vi "UI.VersionCheck.vi"(7 "path":path caption="路径", 8 "错误输入":errorcluster, 10 "Version":string="V1.0.0", 11 "App Name":string="YourAppName.exe") -> (0 "error out":errorcluster caption="错误输出", 2 "OperationCode":i8, 3 "OK?":bool)   [LabVIEW 2012, in "Lib_UEL.ATE.lvlib" / "Lib_App.lvlib"]
uses:
  Lib_App.lvlib
  <vilib>/Utility/config.llb/Read Key (String).vi
  <vilib>/Utility/config.llb/Write Key (String).vi
  <vilib>/Utility/config.llb/NI_LVConfig.lvlib
panel:
  # "OperationCode:\n-255:错误\n-1:运行的不是最新版本\n0:运行版本与版本列表一致\n1:运行版本比版本列表新, 写入最新版本到版本列表\n2:没有在版本列表找到相关版本信息"
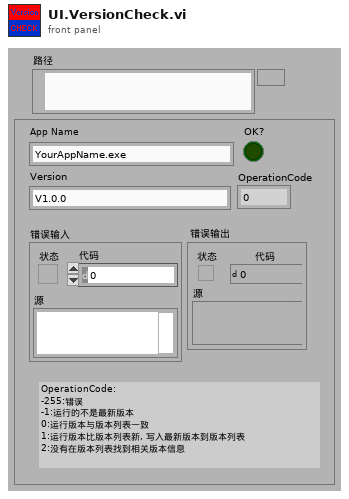
[diagram p1: front panel]
types:
  T1 = typedef "NI_LVConfig.lvlib/Config Data RefNum.ctl" = refnum<k1>
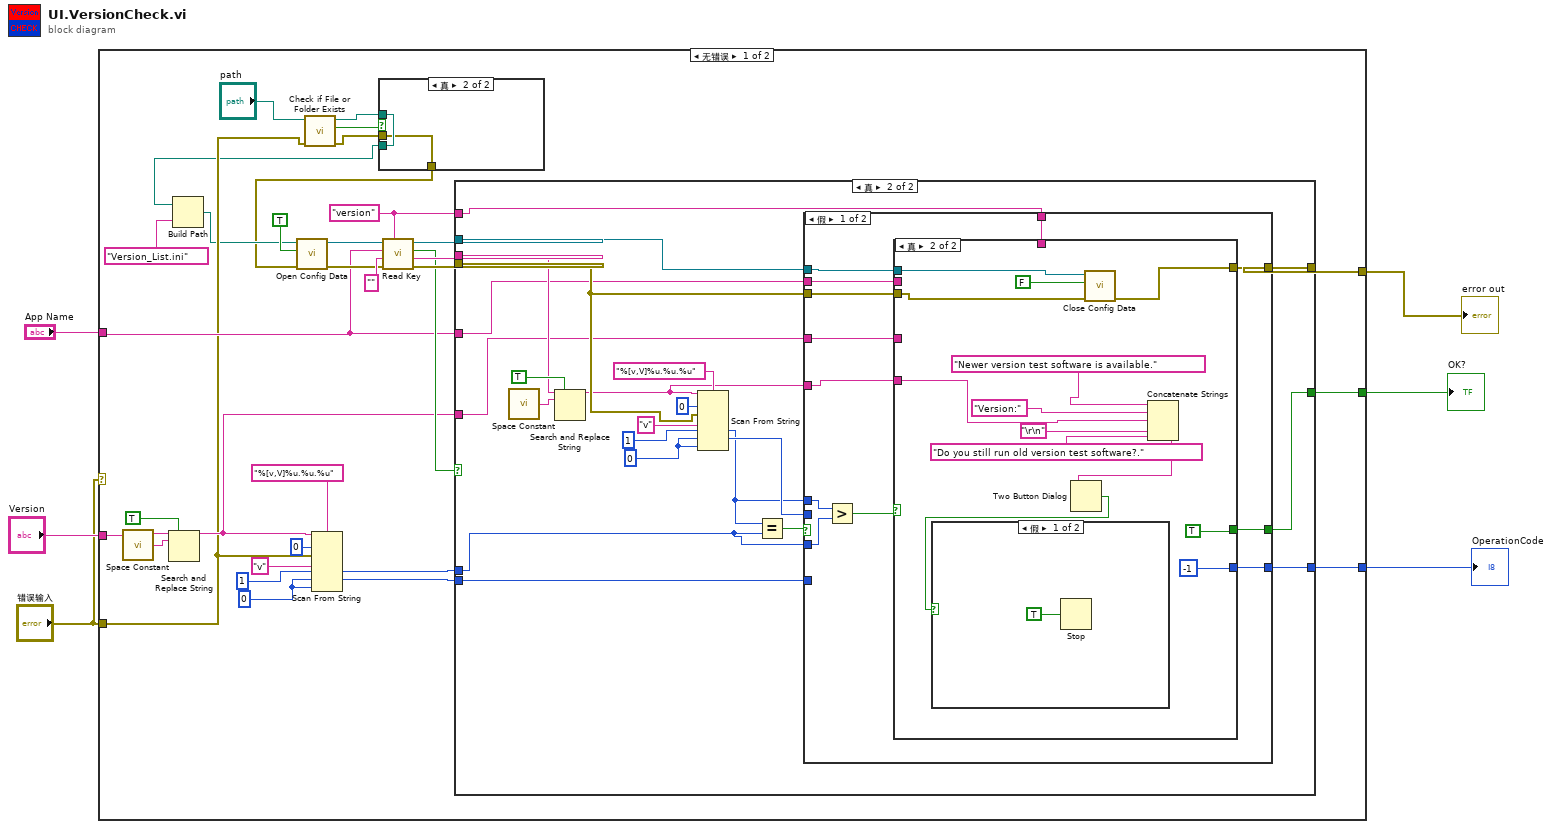
[diagram p0: block diagram]
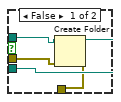
[diagram p2: hidden frame]
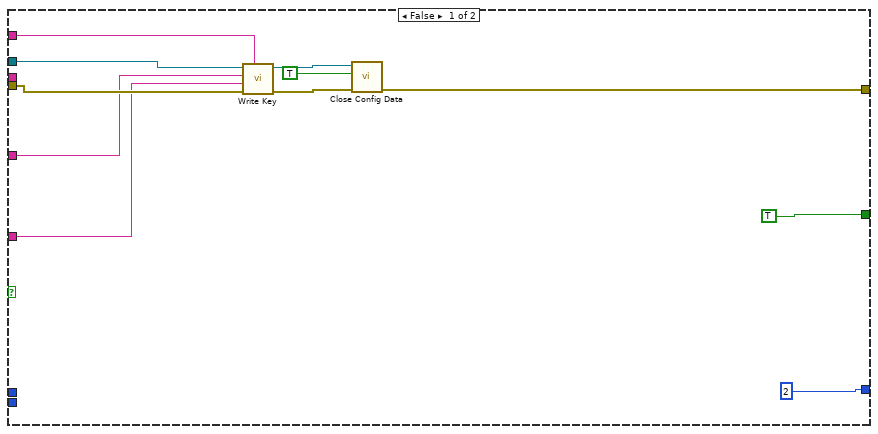
[diagram p3: hidden frame]
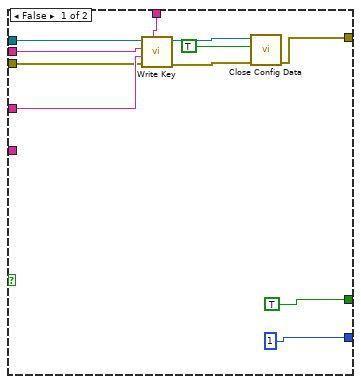
[diagram p4: hidden frame]
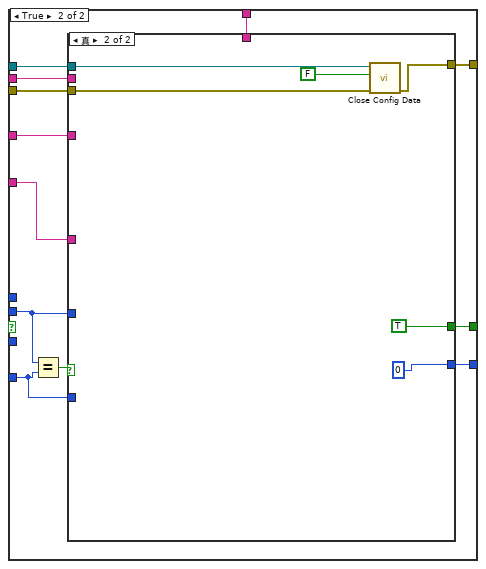
[diagram p6: hidden frame]
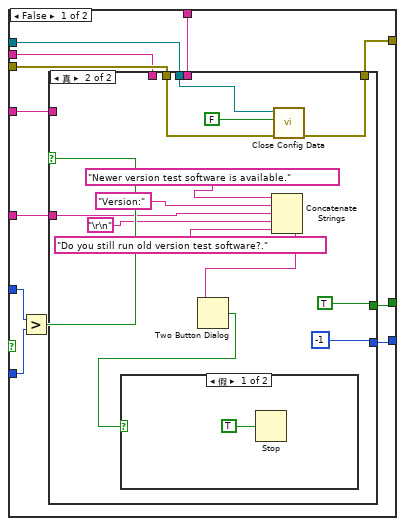
[diagram p7: hidden frame]
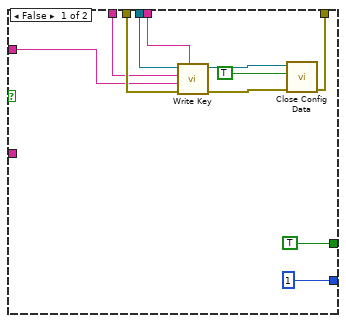
[diagram p8: hidden frame]
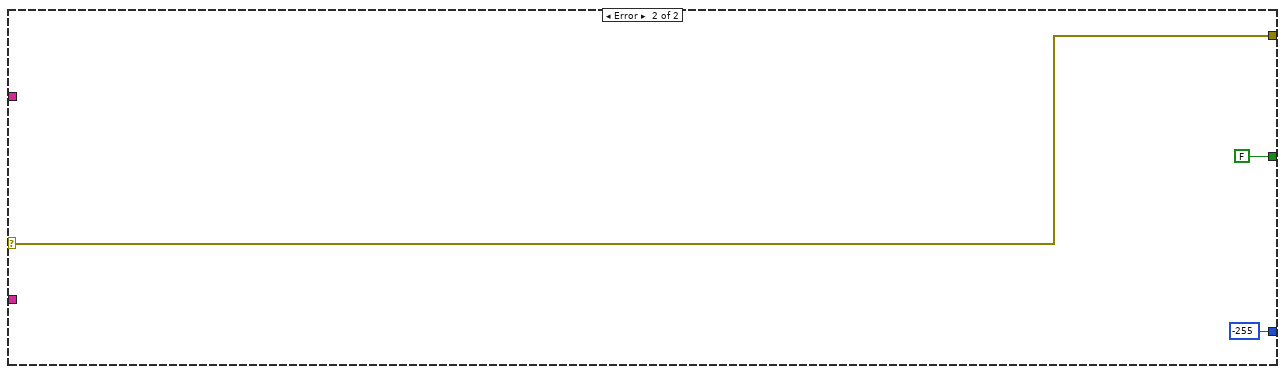
[diagram p10: hidden frame]
diagram:
  n1 = case shown="无错误" "错误输入" {
    selector: "错误输入" -> [_ w173]
    tunnel: "错误输入" -> [w13 _]
    tunnel: "Version" -> [w34 _]
    tunnel: "App Name" -> [w22 _]
    tunnel: [w24 w173] -> w3
    tunnel: [w17 -255] -> w2
    tunnel: [w16 FALSE ("OK?")] -> w1
    frame No Error {
      w20 = "version" ("section")
      w37 = 0 ("默认值 2")
      n2 = call <vilib>:"Space Constant.vi"() -> ("String"=w32:string)
      n3 = Search and Replace String(replace all?=TRUE ("替换全部？(F)"), input string=w34, search string=w32) -> (result string=w21:string)  [unwired: 5 in, 3 out]
      n4 = call <vilib>:"Check if File or Folder Exists.vi"("error in (no error)"=w13, "path"="path") -> ("error out"=w9:errorcluster, "file or folder exists?"=w15:bool, "dup path"=w14:path)  [unwired: 7 in]
      n5 = Scan From String(format string="%[v,V]%u.%u.%u" ("格式字符串"), input string=w21, initial scan location=u32 0 ("初始扫描位置"), error in=w13, default 1="v" ("默认值 1"), default 2=1 ("默认值 1"), default 3=w37, default 4=w37) -> (output 2=w19:i32, output 3=w18:i32)  [unwired: 2 in, 3 out]
      n6 = case shown="真" w15 {
        tunnel: w14 -> [w43 w45]
        tunnel: [w42 w45] -> w11
        tunnel: w9 -> [w41 w44]
        tunnel: [w40 w44] -> w8
        frame False {
          n7 = Create Folder(path (use dialog)=w43, error in=w41) -> (created path=w42:path, error out=w40:errorcluster)  [unwired: 1 in, 1 out]
        }
        frame True {
        }
      }
      n8 = Build Path(base path=w11, name or relative path="Version_List.ini" ("名称或相对路径")) -> (appended path=w10:path)
      n9 = call <vilib>:"Open Config Data.vi"("error in (no error)"=w8, "create file if necessary (T)"=TRUE ("create file if necessary? (T)"), "configuration file path"=w10) -> ("error out"=w27:errorcluster, "refnum"=w30:T1)  [unwired: 6 in, 1 out]
      n10 = call-poly <vilib>:"Read Key.vi"("section"=w20, "error in (no error)"=w27, "default value"="" ("key"), "key"=w22, "refnum"=w30) -> ("error out"=w26:errorcluster, "value"=w28:string, "found?"=w23:bool, "refnum out"=w25:T1)  [unwired: 3 in]
      n11 = case shown="真" w23 {
        tunnel: w28 -> [_ w71]
        tunnel: w26 -> [w56 w64]
        tunnel: w25 -> [w55 w65]
        tunnel: [w48 w63] -> w24
        tunnel: w22 -> [w54 w60]
        tunnel: w21 -> [w53 w61]
        tunnel: w20 -> [w52 w62]
        tunnel: w19 -> [_ w57]
        tunnel: w18 -> [_ w68]
        tunnel: [2 w67] -> w17
        tunnel: [TRUE ("OK?") w66] -> w16
        frame False {
          n12 = call-poly <vilib>:"Write Key.vi"("section"=w52, "error in (no error)"=w56, "value"=w53, "key"=w54, "refnum"=w55) -> ("error out"=w49:errorcluster, "refnum out"=w50:T1)  [unwired: 4 in, 1 out]
          n13 = call <vilib>:"Close Config Data.vi"("error in (no error)"=w49, "write file if changed (T)"=TRUE ("write configuration file? (T)"), "refnum"=w50) -> ("error out"=w48:errorcluster)  [unwired: 7 in, 1 out]
        }
        frame True {
          w74 = 0 ("默认值 2")
          n14 = call <vilib>:"Space Constant.vi"() -> ("String"=w78:string)
          n15 = Search and Replace String(replace all?=TRUE ("替换全部？(F)"), input string=w71, search string=w78) -> (result string=w59:string)  [unwired: 5 in, 3 out]
          n16 = Scan From String(format string="%[v,V]%u.%u.%u" ("格式字符串"), input string=w59, initial scan location=u32 0 ("初始扫描位置"), error in=w64, default 1="v" ("默认值 1"), default 2=1 ("默认值 1"), default 3=w74, default 4=w74) -> (output 2=w58:i32, output 3=w69:i32)  [unwired: 2 in, 3 out]
          n17 = Equal?(x=w58, y=w57) -> (x = y?=w70:bool)
          n18 = case shown="假" w70 {
            tunnel: w69 -> [_ w121]
            tunnel: w68 -> [_ w120]
            tunnel: [w80 w126] -> w67
            tunnel: [w81 w125] -> w66
            tunnel: w65 -> [w89 w124]
            tunnel: w64 -> [w86 w123]
            tunnel: [w85 w122] -> w63
            tunnel: w62 -> [w90 w119]
            tunnel: w61 -> [w87 w118]
            tunnel: w60 -> [w88 w117]
            tunnel: w59 -> [w79 w116]
            tunnel: w58 -> [w84 _]
            tunnel: w57 -> [w83 _]
            frame False {
              n19 = Greater?(x=w84, y=w83) -> (0:w82:bool)
              n20 = case shown="真" w82 {
                tunnel: w90 -> [w98 _]
                tunnel: w89 -> [w97 w104]
                tunnel: w88 -> [w96 _]
                tunnel: w87 -> [w95 _]
                tunnel: w86 -> [w94 w103]
                tunnel: [w93 w102] -> w85
                tunnel: [TRUE ("OK?") TRUE ("OK?")] -> w81
                tunnel: [1 -1] -> w80
                tunnel: w79 -> [_ w108]
                frame False {
                  n21 = call-poly <vilib>:"Write Key.vi"("section"=w98, "error in (no error)"=w94, "value"=w95, "key"=w96, "refnum"=w97) -> ("error out"=w99:errorcluster, "refnum out"=w100:T1)  [unwired: 4 in, 1 out]
                  n22 = call <vilib>:"Close Config Data.vi"("error in (no error)"=w99, "write file if changed (T)"=TRUE ("write configuration file? (T)"), "refnum"=w100) -> ("error out"=w93:errorcluster)  [unwired: 7 in, 1 out]
                }
                frame True {
                  n23 = call <vilib>:"Close Config Data.vi"("error in (no error)"=w103, "write file if changed (T)"=FALSE ("write configuration file? (T)"), "refnum"=w104) -> ("error out"=w102:errorcluster)  [unwired: 7 in, 1 out]
                  n24 = Concatenate Strings("Newer version test software is available." ("消息"), "Version:" ("字符串"), w108, "\r\n", "Do you still run old version test software?." ("消息")) -> (w109:string)
                  n25 = Two Button Dialog(message=w109) -> (T button?=w106:bool)  [unwired: 2 in]
                  n26 = case shown="假" w106 {
                    frame False {
                      n27 = Stop(stop? (T)=TRUE ("停止？(T)")) -> ()
                    }
                    frame True {
                    }
                  }
                }
              }
            }
            frame True {
              n28 = Equal?(x=w121, y=w120) -> (x = y?=w127:bool)
              n29 = case shown="真" w127 {
                tunnel: [w129 0] -> w126
                tunnel: [w130 TRUE ("OK?")] -> w125
                tunnel: w124 -> [w135 w167]
                tunnel: w123 -> [w134 w166]
                tunnel: [w136 w165] -> w122
                tunnel: w121 -> [w139 _]
                tunnel: w120 -> [w138 _]
                tunnel: w119 -> [w137 _]
                tunnel: w118 -> [w133 _]
                tunnel: w117 -> [w132 _]
                tunnel: w116 -> [w128 _]
                frame False {
                  n30 = Greater?(x=w139, y=w138) -> (0:w131:bool)
                  n31 = case shown="真" w131 {
                    tunnel: w137 -> [w147 _]
                    tunnel: [w146 w158] -> w136
                    tunnel: w135 -> [w145 w160]
                    tunnel: w134 -> [w144 w159]
                    tunnel: w133 -> [w143 _]
                    tunnel: w132 -> [w142 _]
                    tunnel: [TRUE ("OK?") TRUE ("OK?")] -> w130
                    tunnel: [1 -1] -> w129
                    tunnel: w128 -> [_ w156]
                    frame False {
                      n32 = call-poly <vilib>:"Write Key.vi"("section"=w147, "error in (no error)"=w144, "value"=w143, "key"=w142, "refnum"=w145) -> ("error out"=w148:errorcluster, "refnum out"=w149:T1)  [unwired: 4 in, 1 out]
                      n33 = call <vilib>:"Close Config Data.vi"("error in (no error)"=w148, "write file if changed (T)"=TRUE ("write configuration file? (T)"), "refnum"=w149) -> ("error out"=w146:errorcluster)  [unwired: 7 in, 1 out]
                    }
                    frame True {
                      n34 = Concatenate Strings("Newer version test software is available." ("消息"), "Version:" ("字符串"), w156, "\r\n", "Do you still run old version test software?." ("消息")) -> (w152:string)
                      n35 = Two Button Dialog(message=w152) -> (T button?=w151:bool)  [unwired: 2 in]
                      n36 = case shown="假" w151 {
                        frame False {
                          n37 = Stop(stop? (T)=TRUE ("停止？(T)")) -> ()
                        }
                        frame True {
                        }
                      }
                      n38 = call <vilib>:"Close Config Data.vi"("error in (no error)"=w159, "write file if changed (T)"=FALSE ("write configuration file? (T)"), "refnum"=w160) -> ("error out"=w158:errorcluster)  [unwired: 7 in, 1 out]
                    }
                  }
                }
                frame True {
                  n39 = call <vilib>:"Close Config Data.vi"("error in (no error)"=w166, "write file if changed (T)"=FALSE ("write configuration file? (T)"), "refnum"=w167) -> ("error out"=w165:errorcluster)  [unwired: 7 in, 1 out]
                }
              }
            }
          }
        }
      }
    }
    frame Error {
    }
  }
  "OK?" <- w1
  "OperationCode" <- w2
  "error out" <- w3
